vi "SinCos0.vi"() -> (8 "SinCos0":refnum<class "SinCos0.lvclass">)   [LabVIEW 2017, in "SinCos0.lvclass"]
uses:
  SinCos0.lvclass
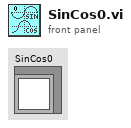
[diagram p1: front panel]
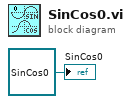
[diagram p0: block diagram]
diagram:
  "SinCos0" <- refnum<class "SinCos0.lvclass"> refnum ("SinCos0.lvclass")
